vi "create_texture_mask.vi"(8 "error in (no error)":errorcluster, 11 "Image Src":T1) -> (0 "error out":errorcluster, 3 "Image":T1(plugin-control))   [LabVIEW 2009]
uses:
  <vilib>/vision/Image Controls.llb/IMAQ Image.ctl
  <vilib>/vision/NI_Vision_Development_Module.lvlib
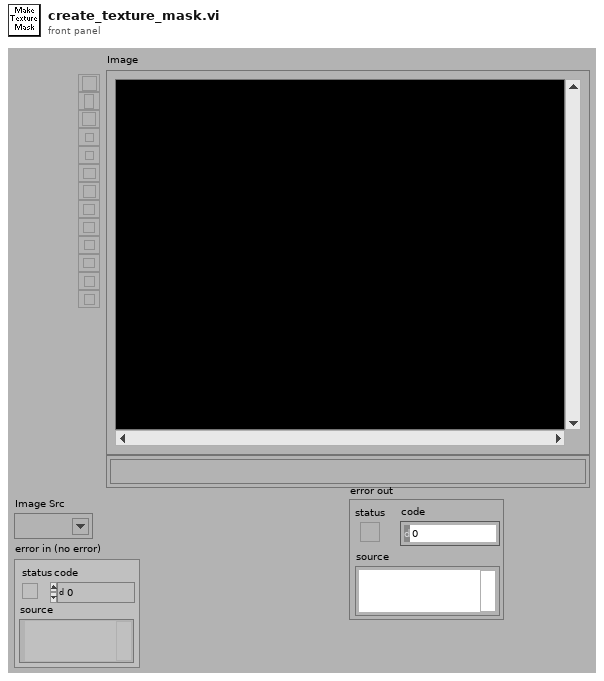
[diagram p1: front panel]
types:
  T1 = typedef "IMAQ Image.ctl" = refnum<image>
  T2 = enum32{"AutoM", "Close", "Dilate", "Erode", "Gradient", "Gradient out", "Gradient in", "Hit miss", "Open", "PClose", "POpen", "Thick", "Thin"}
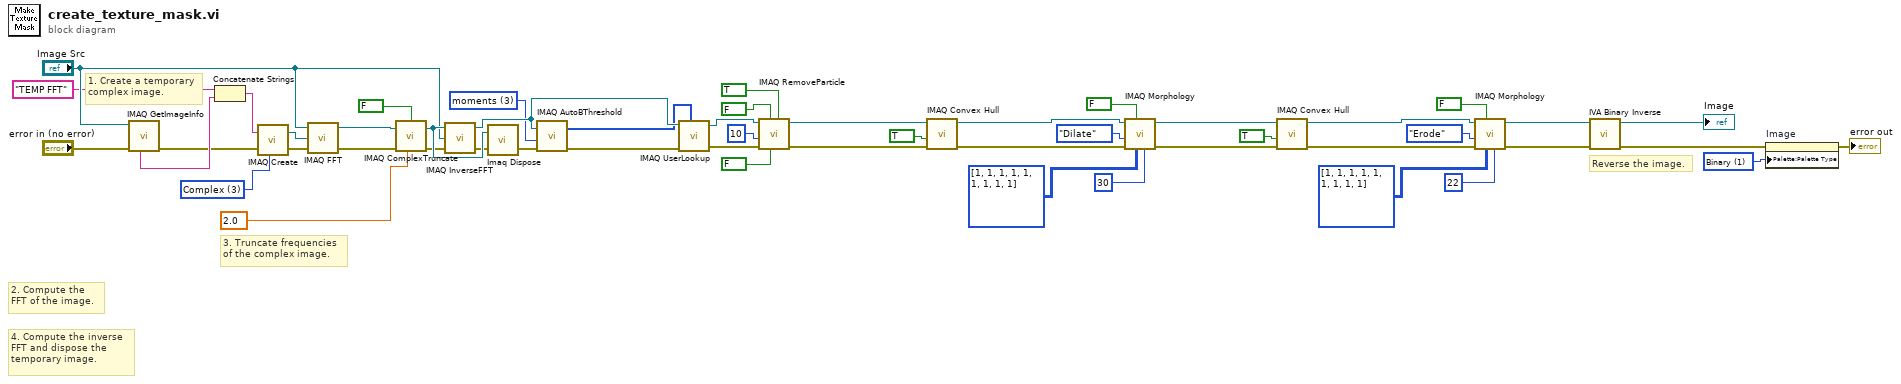
[diagram p0: block diagram]
diagram:
  w9 = 3 items=["clustering", "entropy", "metric", "moments", "inter-class variance"] ("Method")
  w20 = u32 3 items=["8 bits", "16 bits", "Float", "Complex", "RGB", "HSL"] ("Image Type")
  w47 = u32 1 items=["Grayscale", "Binary", "Gradient", "Rainbow", "Temperature", "User Defined"] ("Palette")
  # "3. Truncate frequencies\nof the complex image."
  # "Reverse the image."
  # "4. Compute the inverse\nFFT and dispose the\ntemporary image."
  # "2. Compute the\nFFT of the image."
  # "1. Create a temporary\ncomplex image."
  n1 = call "IMAQ GetImageInfo"("error in (no error)"="error in (no error)", "Image"="Image Src") -> ("error out"=w1:errorcluster, "Image Name"=w4:string)  [unwired: 8 out]
  n2 = Concatenate Strings("TEMP FFT" ("Image Name"), w4) -> (w3:string)
  n3 = call "IMAQ Create"("Image Name"=w3, "Image Type"=w20, "error in (no error)"=w1) -> ("New Image"=w19:T1, "error out"=w13:errorcluster)  [unwired: 1 in, 1 out]
  n4 = call "IMAQ FFT"("error in (no error)"=w13, "Image Dst"=w19, "Image Src"="Image Src") -> ("error out"=w17:errorcluster, "Image Dst Out"=w18:T1)  [unwired: 1 out]
  n5 = call "IMAQ ComplexTruncate"("error in (no error)"=w17, "Truncation Frequency %"=sgl 2.0, "Image Src"=w18, "Low pass/High pass (Low pass)"=FALSE) -> ("error out"=w15:errorcluster, "Image Dst Out"=w16:T1)  [unwired: 1 in, 2 out]
  n6 = call "IMAQ InverseFFT"("error in (no error)"=w15, "Image Dst"="Image Src", "Image Src"=w16) -> ("error out"=w14:errorcluster, "Image Dst Out"=w51:T1)  [unwired: 1 out]
  n7 = call "Imaq Dispose"("Image"=w16, "error in (no error)"=w14) -> ("error out"=w50:errorcluster)  [unwired: 1 in, 3 out]
  n8 = call "IMAQ AutoBThreshold"("error in (no error)"=w50, "Method"=w9, "Image"=w51) -> ("error out"=w7:errorcluster, "Lookup Table"=w8:i16[])  [unwired: 1 in, 3 out]
  n9 = call "IMAQ UserLookup"("Image Src"=w51, "Lookup Table"=w8, "error in (no error)"=w7) -> ("Image Dst Out"=w10:T1, "error out"=w29:errorcluster)  [unwired: 2 in, 2 out]
  n10 = call "IMAQ RemoveParticle"("Connectivity 4/8 (8)"=TRUE, "Low Pass/High Pass (Low)"=FALSE, "Square/Hexa (Square)"=FALSE, "error in (no error)"=w29, "Number of Erosion"=10, "Image Src"=w10) -> ("error out"=w40:errorcluster, "Image Dst Out"=w41:T1)  [unwired: 1 in, 3 out]
  n11 = call "IMAQ Convex Hull"("error in (no error)"=w40, "Connectivity 4/8 (8)"=TRUE, "Image Src"=w41) -> ("error out"=w38:errorcluster, "Image Dst Out"=w37:T1)  [unwired: 1 in, 6 out]
  n12 = call "IMAQ Morphology"("Number of iterations (1)"=30, "Structuring Element"=i32[][] [[1, 1, 1], [1, 1, 1], [1, 1, 1]], "Square/Hexa (Square)"=FALSE, "error in (no error)"=w38, "Operation"=T2."Dilate", "Image Src"=w37) -> ("error out"=w31:errorcluster, "Image Dst Out"=w32:T1)  [unwired: 1 in, 3 out]
  n13 = call "IMAQ Convex Hull"("error in (no error)"=w31, "Connectivity 4/8 (8)"=TRUE, "Image Src"=w32) -> ("error out"=w24:errorcluster, "Image Dst Out"=w23:T1)  [unwired: 1 in, 6 out]
  n14 = call "IMAQ Morphology"("Number of iterations (1)"=22, "Structuring Element"=i32[][] [[1, 1, 1], [1, 1, 1], [1, 1, 1]], "Square/Hexa (Square)"=FALSE, "error in (no error)"=w24, "Operation"=T2."Erode", "Image Src"=w23) -> ("error out"=w21:errorcluster, "Image Dst Out"=w22:T1)  [unwired: 1 in, 3 out]
  n15 = call <vilib>:"IVA Binary Inverse.vi"("error in (no error)"=w21, "Image In"=w22) -> ("error out"=w48:errorcluster, "Image Out"=→"Image":T1)  [unwired: 8 out]
  n16 = property on="Image" class="ImageControl"(error in=w48, "Palette:Palette Type"=w47) -> (error out=→"error out":errorcluster)  [unwired: 1 in, 1 out]
